vi "ExtractLeftovers.vi"(9 "Hits":T1(array[cluster]), 10 "Oldest allowable hit":u64) -> (3 "Leftovers new":T1(array[cluster]))   [LabVIEW 2016]
uses:
  Global Variables/System info.vi
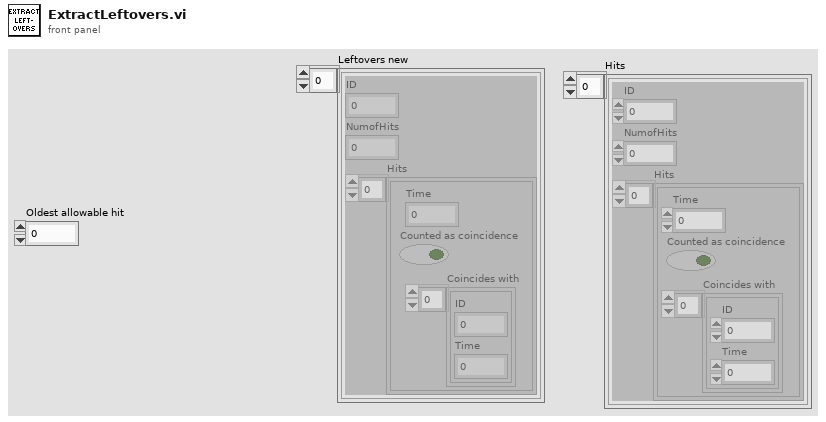
[diagram p1: front panel]
types:
  T1 = cluster{"ID":i8, "NumofHits":i32, "Hits":cluster{"Time":u64, "Counted as coincidence":bool, "Coincides with":cluster{"ID":i8, "Time":u64}[]}[]}[]
  T2 = cluster{"ID":i8, "NumofHits":i32, "Hits":cluster{"Time":i64, "Counted as coincidence":bool, "Coincides with":cluster{"ID":i8, "Time":i64}[]}[]}[]
  T3 = cluster{"Time":i64, "Counted as coincidence":bool, "Coincides with":cluster{"ID":i8, "Time":i64}[]}[]
  T4 = cluster{"Time":u64, "Counted as coincidence":bool, "Coincides with":cluster{"ID":i8, "Time":u64}[]}[]
  T5 = cluster{"Time":u64, "Counted as coincidence":bool, "Coincides with":cluster{"ID":i8, "Time":u64}[]}
  T6 = cluster{"ID":i8, "NumofHits":i32, "Hits":cluster{"Time":i64, "Counted as coincidence":bool, "Coincides with":cluster{"ID":i8, "Time":i64}[]}[]}
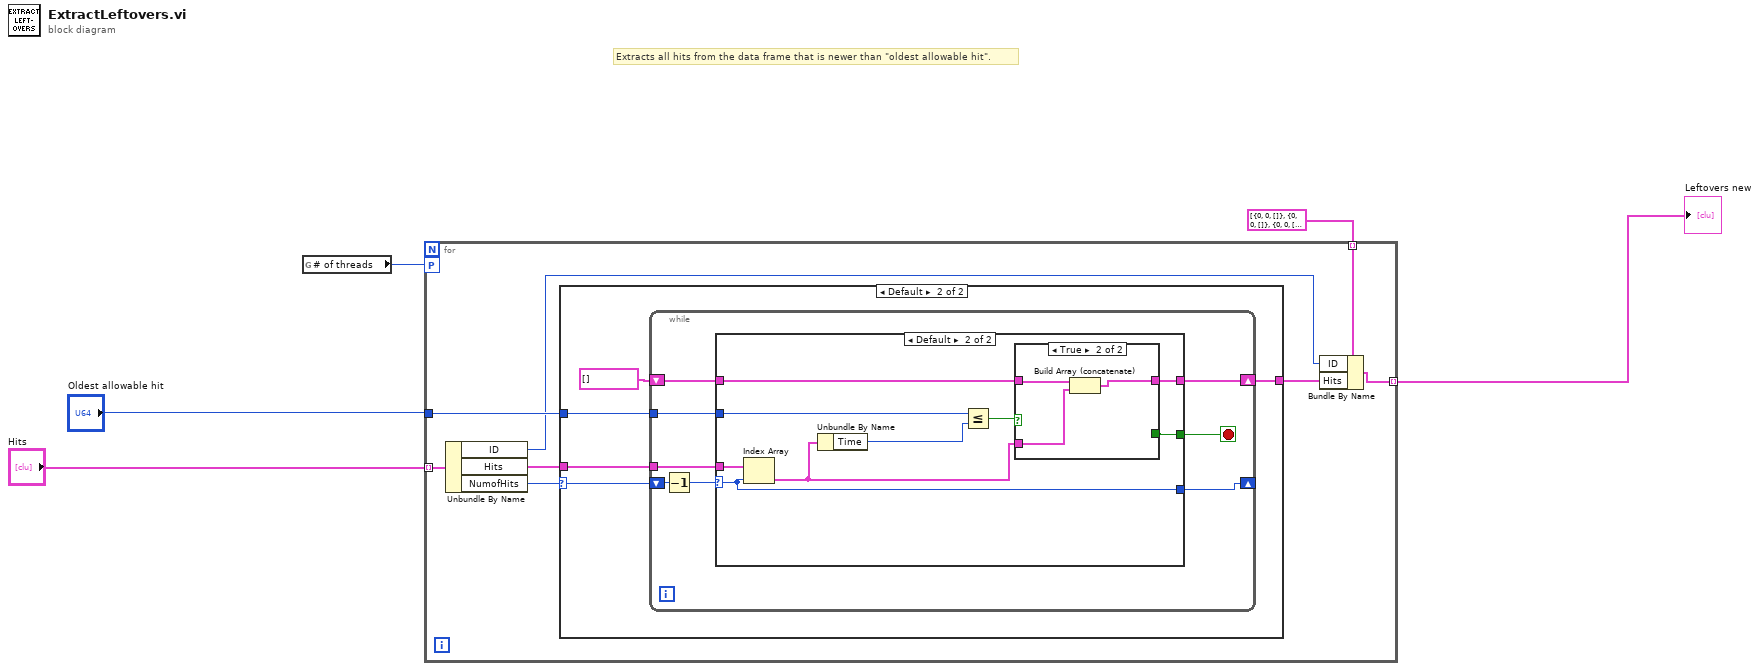
[diagram p0: block diagram]
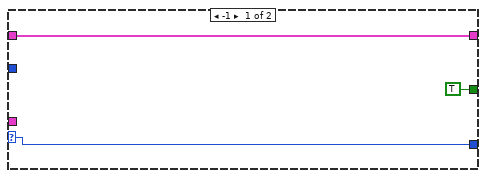
[diagram p3: hidden frame]
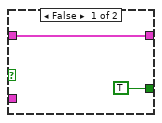
[diagram p4: hidden frame]
diagram:
  # "Extracts all hits from the data frame that is newer than \"oldest allowable hit\"."
  n1 = global read "System info.vi" "# of threads"() -> (w1:i32)
  n2 = for {
    tunnel: "Hits" -> [w13] mode=indexing
    tunnel: "Oldest allowable hit" -> [w11]
    tunnel: T2 [{"ID"=0, "NumofHits"=0, "Hits"=[]}, {"ID"=0, "NumofHits"=0, "Hits"=[]}, {"ID"=0, "NumofHits"=0, "Hits"=[]}, {"ID"=0, "NumofHits"=0, "Hits"=[]}, {"ID"=0, "NumofHits"=0, "Hits"=[]}] ("Leftovers old") -> [w9] mode=indexing
    tunnel: [w7] -> w4 mode=indexing
    workers-P: w1 -> [_]
    n3 = Unbundle By Name(w13) -> ("ID"=w6:i8, "Hits"=w12:T4, "NumofHits"=w10:i32)
    n4 = case shown="Default" w10 {
      selector: w10 -> [_ w16]
      tunnel: w12 -> [_ w18]
      tunnel: w11 -> [_ w17]
      tunnel: [_ w14] -> w8
      frame 0 {
      }
      frame Default {
        n5 = while {
          tunnel: w18 -> [w26]
          tunnel: w17 -> [w24]
          shift-right: [w19] -> _
          shift-left: w16 -> [w25]
          shift-right: [w22] -> w14
          shift-left: T3 [] -> [w23]
          stop <- w21 stop-if-true
          n6 = Decrement(x=w25) -> (x-1=w20:i32)
          n7 = case shown="Default" w20 {
            selector: w20 -> [w27 w30]
            tunnel: w26 -> [_ w38]
            tunnel: w24 -> [_ w37]
            tunnel: w23 -> [w28 w35]
            tunnel: [w28 w34] -> w22
            tunnel: [TRUE w33] -> w21
            tunnel: [w27 w30] -> w19
            frame -1 {
            }
            frame Default {
              n8 = Index Array(array=w38, index=w30) -> (element=w31:T5)
              n9 = Unbundle By Name(w31) -> ("Time"=w32:u64)
              n10 = Less Or Equal?(x=w37, y=w32) -> (x <= y?=w36:bool)
              n11 = case shown="True" w36 {
                tunnel: w35 -> [w40 w43]
                tunnel: w31 -> [_ w42]
                tunnel: [w40 w41] -> w34
                tunnel: [TRUE _] -> w33
                frame False {
                }
                frame True {
                  n12 = Build Array (concatenate)(w43, w42) -> (w41:T4)
                }
              }
            }
          }
        }
      }
    }
    n13 = Bundle By Name(cluster=w9, "ID"=w6, "Hits"=w8) -> (w7:T6)
  }
  "Leftovers new" <- w4
